vi "HumiCov.vi"(11 "Input x":dbl) -> (3 "Humidity":dbl)   [LabVIEW 2011]
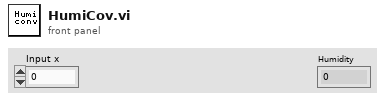
[diagram p1: front panel]
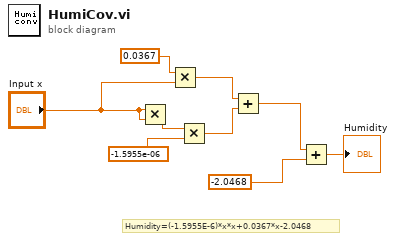
[diagram p0: block diagram]
diagram:
  # "Humidity=(-1.5955E-6)*x*x+0.0367*x-2.0468"
  n1 = Multiply(x="Input x", y="Input x") -> (x*y=w8:dbl)
  n2 = Multiply(x=0.0367, y="Input x") -> (x*y=w6:dbl)
  n3 = Multiply(x=w8, y=-1.5955e-06) -> (x*y=w5:dbl)
  n4 = Add(x=w6, y=w5) -> (x+y=w4:dbl)
  n5 = Add(x=w4, y=-2.0468) -> (x+y=→"Humidity":dbl)
